vi "表换线提示.vi"(8 "error in (no error)":errorcluster caption="错误输入（无错误）", 11 "34461A 输入":refnum<class "34461A.lvclass">) -> (0 "error out":errorcluster caption="错误输出", 3 "34461A 输出":refnum<class "34461A.lvclass">)   [LabVIEW 2020, in "34461A.lvlib" / "34461A.lvclass"]
uses:
  34461A.lvclass
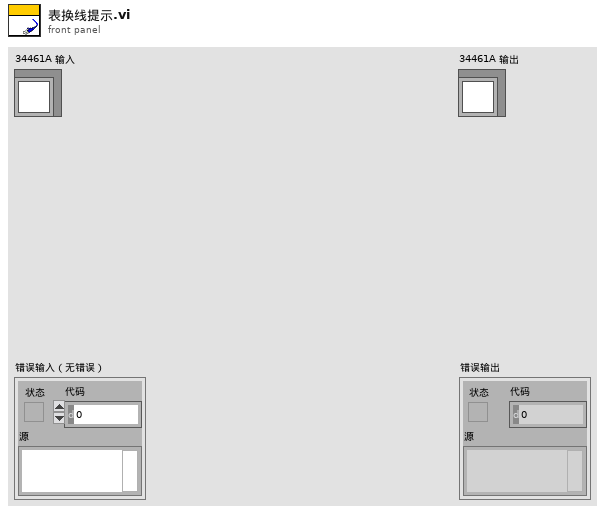
[diagram p1: front panel]
types:
  T1 = enum16{"DC Voltage", "AC Voltage", "Resistance", "DC Current", "AC Current"}
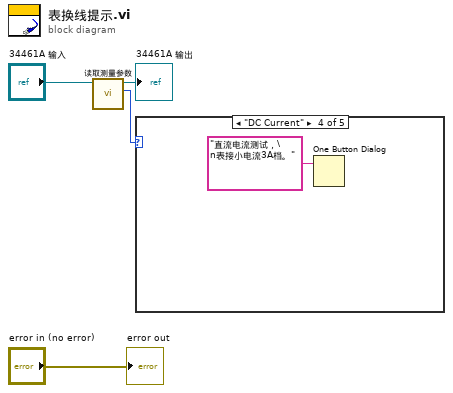
[diagram p0: block diagram]
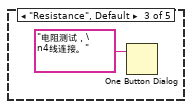
[diagram p4: hidden frame]
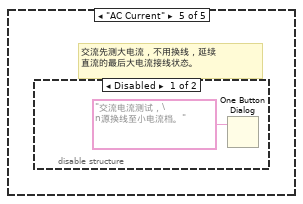
[diagram p5: hidden frame]
diagram:
  n1 = call "读取测量参数.vi"("数字多用表接口输入"="34461A 输入") -> ("测量参数"=w3:T1, "数字多用表接口输出"=→"34461A 输出":refnum<class "34461A.lvclass">)  [unwired: 8 in, 1 out]
  n2 = case shown="\"DC Current\"" w3 {
    frame "DC Voltage" {
    }
    frame "AC Voltage" {
    }
    frame "Resistance", Default {
      n3 = One Button Dialog(message="电阻测试，\n4线连接。") -> ()  [unwired: 1 in, 1 out]
    }
    frame "DC Current" {
      n4 = One Button Dialog(message="直流电流测试，\n表接小电流3A档。") -> ()  [unwired: 1 in, 1 out]
    }
    frame "AC Current" {
      # "交流先测大电流，不用换线，延续\n直流的最后大电流接线状态。"
      n5 = disable-structure shown="Disabled" {
        frame Disabled {
          n6 = One Button Dialog(message="交流电流测试，\n源换线至小电流档。") -> ()  [unwired: 1 in, 1 out]
        }
        frame Enabled {
        }
      }
    }
  }
  "error out" <- "error in (no error)"
